vi "Set VI Properties.vi"(9 "Front Panel Controls":T1, 11 "Item Data":refnum<class "Item.lvclass">[](array[class])) -> (3 "Item Data out":refnum<class "Item.lvclass">[](array[class]))   [LabVIEW 2020, in "VI Properties Editor.lvlib"]
doc: "Sets all new VI properties of a VI within <B>Item Data</B> based on <B>Front Panel Controls</B>."
uses:
  VI Properties Editor.lvlib
  Classes/Item/Item.lvclass
  CTLs/Main Front Panel Controls.ctl
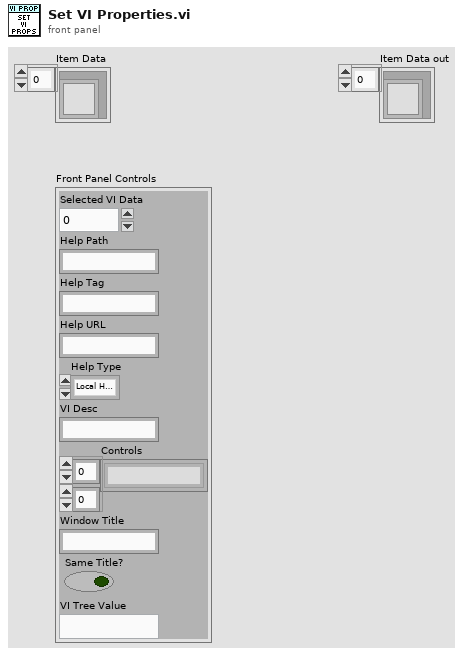
[diagram p1: front panel]
types:
  T1 = typedef "VI Properties Editor.lvlib/Main Front Panel Controls.ctl" = cluster{"Selected VI Data":i32, "Help Path":string, "Help Tag":string, "Help URL":string, "Help Type":enum16{"Local Help File", "Web-based Help"}, "VI Desc":string, "Controls":string[][], "Window Title":string, "Same Title?":bool, "VI Tree Value":string}
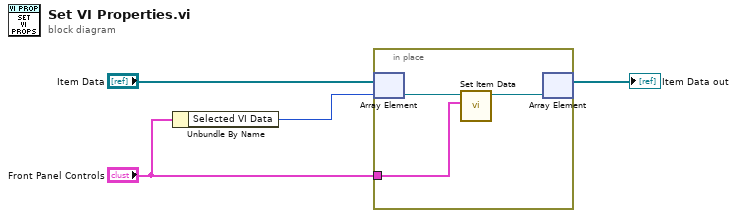
[diagram p0: block diagram]
diagram:
  n1 = Unbundle By Name("Front Panel Controls") -> ("Selected VI Data"=w2:i32)
  n2 = in-place {
    in-place-border: "Front Panel Controls" -> [w5]
    n3 = in-place-array #1("Item Data", w2) -> (w7:refnum<class "Item.lvclass">)
    n4 = call-dynamic "Set Item Data.vi"("Front Panel Controls"=w5, "Item in"=w7) -> ("Item out"=w6:refnum<class "Item.lvclass">)  [unwired: 8 in, 1 out]
    n5 = in-place-array #1(w6) -> (→"Item Data out":refnum<class "Item.lvclass">[])  [unwired: 1 out]
  }
